vi "DSF.Engine.Interface.RT FIFO.Delete.vi"   [LabVIEW 2017, in "Data Sharing Framework Engine.lvlib" / "DSF.Engine.Interface.lvclass"]
uses:
  DSF.Engine.Interface.lvclass
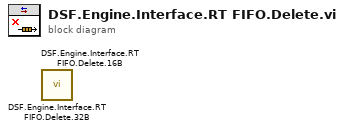
[diagram p0: block diagram]
diagram:
  n1 = call "DSF.Engine.Interface.RT FIFO.Delete.32B.vi"() -> ()  [unwired: 11 in, 1 out]
  n2 = call "DSF.Engine.Interface.RT FIFO.Delete.16B.vi"() -> ()  [unwired: 11 in, 1 out]
